vi "Size Front Panel Objects.vi"(8 "error out":errorcluster, 11 "User Interface References":T1) -> (0 "error IO 2":errorcluster, 3 "User Interface References Out":T1)   [LabVIEW 2010]
uses:
  <vilib>/Utility/config.llb/NI_LVConfig.lvlib
  <vilib>/Utility/config.llb/Read Key (I32).vi
  <vilib>/Utility/config.llb/Config Data RefNum.ctl
  Sliding Menu Type Definitions/User Interface Type Definitions.ctl
  Menu Buttons_old/Menu Button XControl/Menu Button XControl.xctl
  Avatar2/Avatar SubVIs/Main Type Definitions/UI Picture Containers.ctl
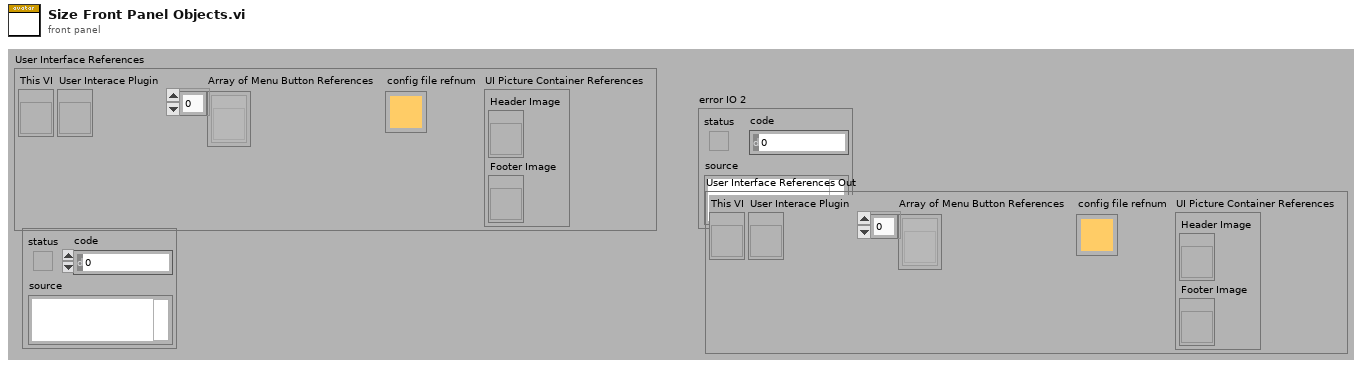
[diagram p1: front panel]
types:
  T1 = typedef "User Interface Type Definitions.ctl" = cluster{"This VI":refnum<vi>, "User Interace Plugin":refnum<vi>, "Array of Menu Button References":refnum<vi>[], "config file refnum":T2, "UI Picture Container References":T3}
  T2 = typedef "NI_LVConfig.lvlib/Config Data RefNum.ctl" = refnum<k1>
  T3 = typedef "UI Picture Containers.ctl" = cluster{"Header Image":refnum<vi>, "Footer Image":refnum<vi>}
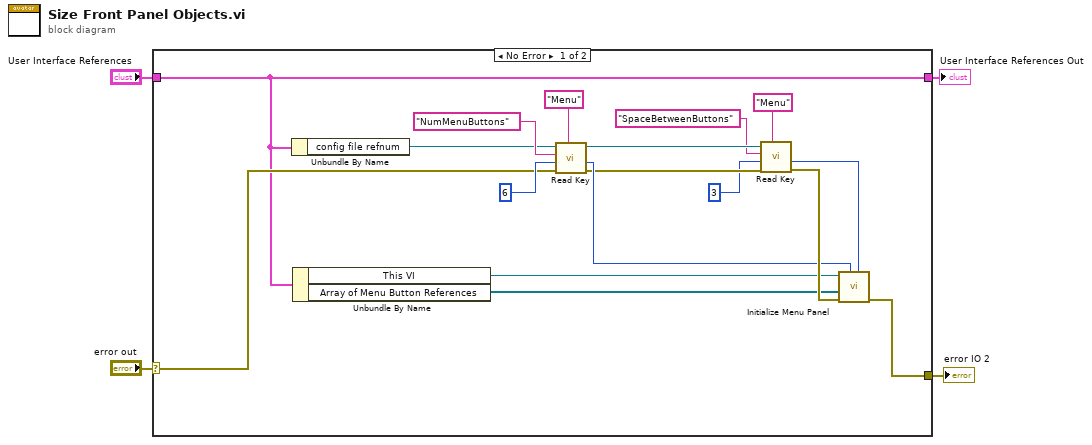
[diagram p0: block diagram]
diagram:
  n1 = case shown="No Error" "error out" {
    selector: "error out" -> [w6 w22]
    tunnel: "User Interface References" -> [w5 _]
    tunnel: [w9 w22] -> w3
    tunnel: [w5 _] -> w1
    frame No Error {
      n2 = Unbundle By Name(w5) -> ("config file refnum"=w15:T2)
      n3 = Unbundle By Name(w5) -> ("This VI"=w7:refnum<vi>, "Array of Menu Button References"=w8:refnum<vi>[])
      n4 = call-poly <vilib>:"Read Key.vi"("section"="Menu", "error in (no error)"=w6, "default value"=6, "key"="NumMenuButtons", "refnum"=w15) -> ("error out"=w19:errorcluster, "value"=w20:i32, "refnum out"=w18:T2)  [unwired: 3 in, 1 out]
      n5 = call-poly <vilib>:"Read Key.vi"("section"="Menu", "error in (no error)"=w19, "default value"=3, "key"="SpaceBetweenButtons", "refnum"=w18) -> ("error out"=w21:errorcluster, "value"=w13:i32)  [unwired: 3 in, 2 out]
      n6 = call "Initialize Menu Panel.vi"("Space Between Panels"=w13, "Number of Panels to Show at the Same Time"=w20, "error in"=w21, "Array of Menu Button References"=w8, "This VI"=w7) -> ("error IO 2"=w9:errorcluster)  [unwired: 5 in, 1 out]
    }
    frame Error {
    }
  }
  "error IO 2" <- w3
  "User Interface References Out" <- w1
